vi "Read value.vi"(8 "error in (no error)":errorcluster, 11 "MCP4725 in":refnum<class "MCP4725.lvclass">) -> (0 "error out":errorcluster, 2 "value":string, 3 "MCP4725 out":refnum<class "MCP4725.lvclass">)   [LabVIEW 2014, in "LabVIEW Universal Transcriptor MCP4725.lvlib" / "MCP4725.lvclass"]
uses:
  MCP4725.lvclass
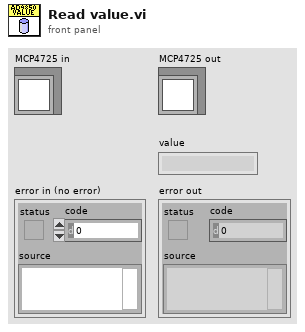
[diagram p1: front panel]
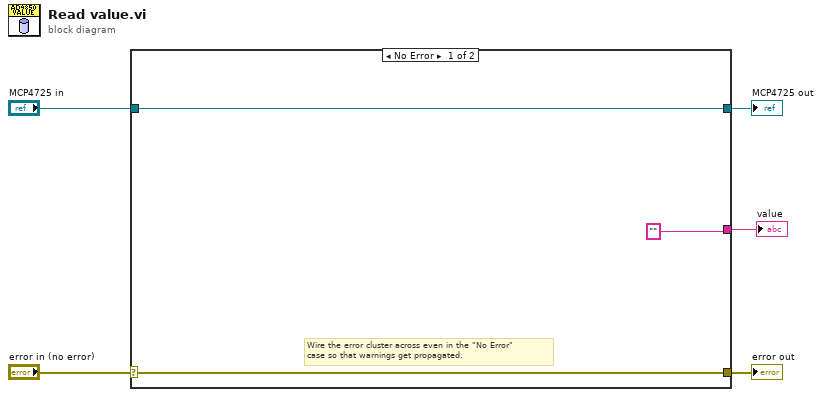
[diagram p0: block diagram]
diagram:
  n1 = case shown="No Error" "error in (no error)" {
    selector: "error in (no error)" -> [w7 w10]
    tunnel: [w7 w10] -> w4
    tunnel: [w8 w9] -> w2
    tunnel: "MCP4725 in" -> [w8 w9]
    tunnel: ["" _] -> w1
    frame No Error {
      # "Wire the error cluster across even in the \"No Error\"\ncase so that warnings get propagated."
    }
    frame Error {
    }
  }
  "error out" <- w4
  "MCP4725 out" <- w2
  "value" <- w1
